vi "MousePosToFPWinBound.vi"(6 "Y offset":i32, 7 "axis info":T2, 8 "Active Box":T1, 9 "Height":i32, 10 "X offset":i32, 11 "Width":i32) -> (1 "Output Bounds":T1)   [LabVIEW 2023, in "FolloWin.lvclass"]
doc: "Calculate FolloWin window Bounds from parameters and mouse position."
uses:
  FolloWin.lvclass
  <vilib>/Utility/miscctls.llb/LVRectTypeDef.ctl
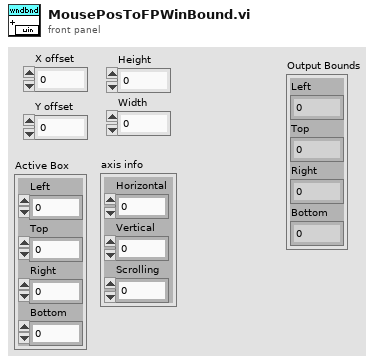
[diagram p1: front panel]
types:
  T1 = typedef "LVRectTypeDef.ctl" = cluster{"Left":i16, "Top":i16, "Right":i16, "Bottom":i16}
  T2 = cluster{"Horizontal":i32, "Vertical":i32, "Scrolling":i32}
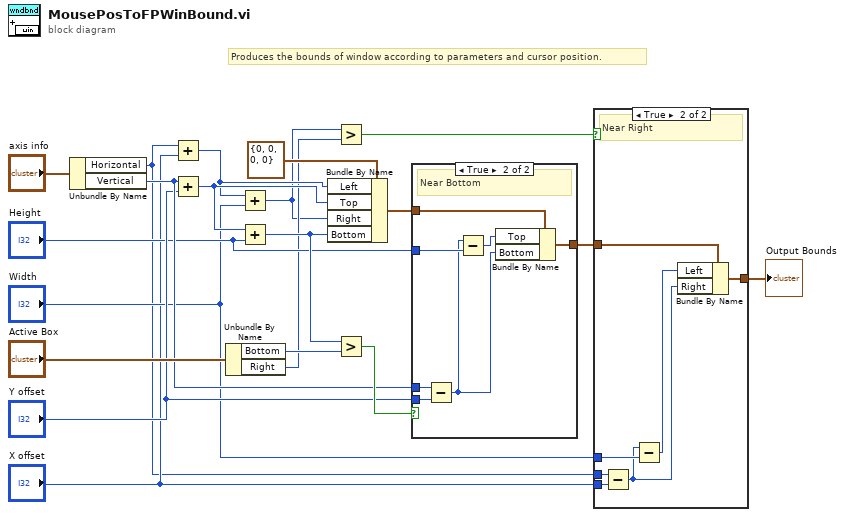
[diagram p0: block diagram]
diagram:
  # "Produces the bounds of window according to parameters and cursor position."
  n1 = Unbundle By Name("axis info") -> ("Horizontal"=w2:i32, "Vertical"=w11:i32)
  n2 = Add(x=w2, y="X offset") -> (x+y=w19:i32)
  n3 = Add(x=w11, y="Y offset") -> (x+y=w20:i32)
  n4 = Unbundle By Name("Active Box") -> ("Bottom"=w15:i16, "Right"=w7:i16)
  n5 = Add(x=w19, y="Width") -> (x+y=w6:i32)
  n6 = Add(x=w20, y="Height") -> (x+y=w14:i32)
  n7 = Bundle By Name(cluster=T1 {"Left"=0, "Top"=0, "Right"=0, "Bottom"=0} ("input cluster"), "Left"=w19, "Top"=w20, "Right"=w6, "Bottom"=w14) -> (w12:T1)
  n8 = Greater?(x=w6, y=w7) -> (0:w8:bool)
  n9 = Greater?(x=w14, y=w15) -> (0:w13:bool)
  n10 = case shown="True" w13 {
    tunnel: w12 -> [w21 w28]
    tunnel: [w21 w27] -> w5
    tunnel: w11 -> [_ w26]
    tunnel: "Y offset" -> [_ w25]
    tunnel: "Height" -> [_ w24]
    frame False {
    }
    frame True {
      # "Near Bottom"
      n11 = Subtract(x=w26, y=w25) -> (x-y=w22:i32)
      n12 = Subtract(x=w22, y=w24) -> (x-y=w23:i32)
      n13 = Bundle By Name(cluster=w28, "Top"=w23, "Bottom"=w22) -> (w27:T1)
    }
  }
  n14 = case shown="True" w8 {
    tunnel: w5 -> [w29 w36]
    tunnel: [w29 w35] -> w1
    tunnel: w2 -> [_ w31]
    tunnel: "X offset" -> [_ w34]
    tunnel: "Width" -> [_ w33]
    frame False {
    }
    frame True {
      # "Near Right"
      n15 = Subtract(x=w31, y=w34) -> (x-y=w30:i32)
      n16 = Subtract(x=w30, y=w33) -> (x-y=w32:i32)
      n17 = Bundle By Name(cluster=w36, "Left"=w32, "Right"=w30) -> (w35:T1)
    }
  }
  "Output Bounds" <- w1
